vi "macro_Digital_OrMany.vi"   [LabVIEW 2019, in "Trajectory_Library.lvlib"]
uses:
  Trajectory_Library.lvlib
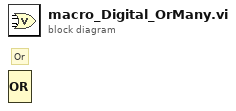
[diagram p0: block diagram]
diagram:
  # "Or"
  n1 = Compound Arithmetic op=OR() -> ()  [unwired: 4 in, 1 out]
